vi "Initialize.vi"(5 "TCP Configuration":T1, 7 "Serial Port":refnum<visa-resource-name>="N/A", 8 "Error In":errorcluster, 10 "Interface":T2, 11 "Platform":T7) -> (0 "Error Out":errorcluster, 2 "Device Name":string, 3 "LINX Ref":T3)   [LabVIEW 2013, in "LVH-LINX.lvlib"]
doc: "Initialize a connection to a LINX device."
uses:
  <vilib>/LabVIEW Hacker/LINX/LVH-LINX.lvlib
  <vilib>/LabVIEW Hacker/LINX/Private/Type Defs/User Platform.ctl
  <vilib>/LabVIEW Hacker/LINX/Private/Type Defs/LINX Ref.ctl
  <vilib>/LabVIEW Hacker/LINX/Private/Type Defs/Platform.ctl
  <vilib>/LabVIEW Hacker/LINX/Private/Type Defs/Interface.ctl
  <vilib>/LabVIEW Hacker/LINX/Private/Device/Type Defs/LINX Device Config.ctl
  <vilib>/LabVIEW Hacker/LINX/Private/Device/Type Defs/TCP Config.ctl
  <vilib>/LabVIEW Hacker/LINX/Private/Type Defs/Device Family.ctl
  <vilib>/LabVIEW Hacker/LINX/Private/Type Defs/Channel FGV States.ctl
  <vilib>/LabVIEW Hacker/LINX/Private/Device/Device.lvlib
  <vilib>/LabVIEW Hacker/LINX/Private/Type Defs/Devices - NI.ctl
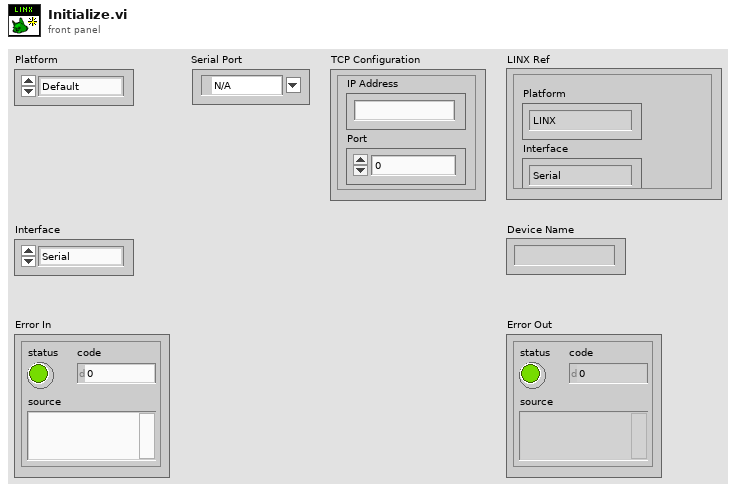
[diagram p1: front panel]
types:
  T1 = typedef "LVH-LINX.lvlib/Device.lvlib/TCP Config.ctl" = cluster{"IP Address":string, "Port":u16}
  T2 = typedef "LVH-LINX.lvlib/Interface.ctl" = enum16{"Serial", "TCP"}
  T3 = typedef "LVH-LINX.lvlib/LINX Ref.ctl" = cluster{"Platform":T4, "Interface":T2, "LINX Device Config":T5}
  T4 = typedef "LVH-LINX.lvlib/Platform.ctl" = enum16{"LINX", "myRIO"}
  T5 = typedef "LVH-LINX.lvlib/Device.lvlib/LINX Device Config.ctl" = cluster{"Interface":T2, "COM Port":refnum<visa-resource-name>, "TCP Configuration":T1, "Device Family":T6, "Device ID":u8, "Device Name":string, "TCP Ref":refnum<k5>}
  T6 = typedef "LVH-LINX.lvlib/Device Family.ctl" = enum8{"National Instruments", "Digilent", "Arduino"}
  T7 = typedef "LVH-LINX.lvlib/User Platform.ctl" = enum16{"Default", "LINX", "myRIO"}
  T8 = typedef "LVH-LINX.lvlib/Devices - NI.ctl" = enum16{"myRIO-1900", "myRIO-1950"}
  T9 = typedef "LVH-LINX.lvlib/Channel FGV States.ctl" = enum16{"Initialize", "Get", "Set"}
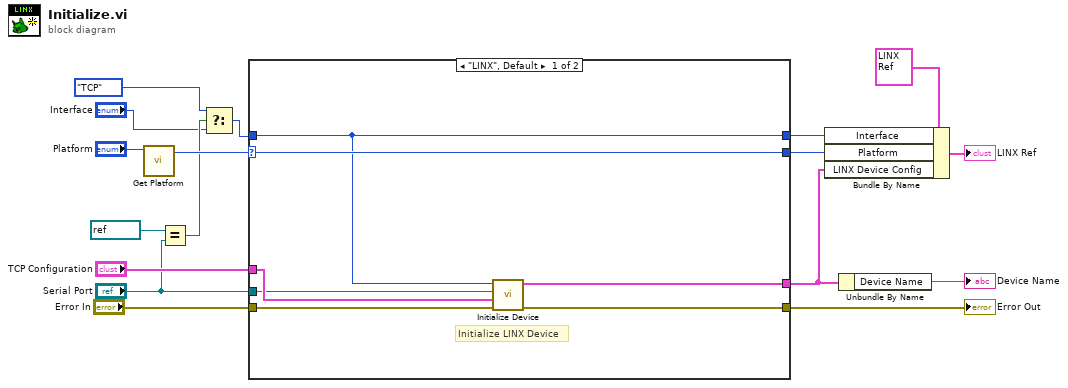
[diagram p0: block diagram]
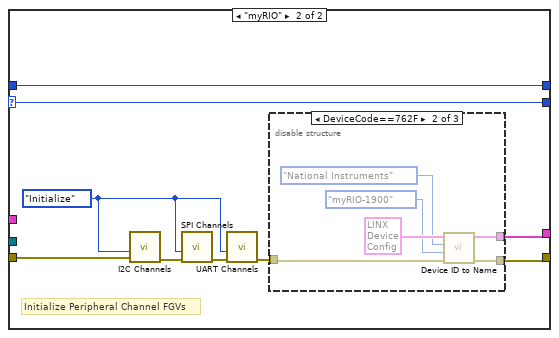
[diagram p2: hidden frame]
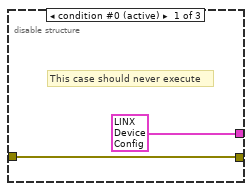
[diagram p3: hidden frame]
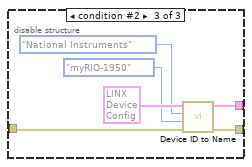
[diagram p4: hidden frame]
diagram:
  n1 = call <vilib>:"Get Platform.vi"("Platform"="Platform") -> ("Platform"=w15:T4)  [unwired: 10 in]
  n2 = Equal?(x=refnum<visa-resource-name> "N/A", y="Serial Port") -> (x = y?=w4:bool)
  n3 = Select(t=Interface."TCP" ("f"), s=w4, f="Interface") -> (s? t:f=w3:T2)
  n4 = case shown="\"LINX\", Default" w15 {
    selector: w15 -> [w24 w33]
    tunnel: [w21 w30] -> w8
    tunnel: [w22 w29] -> w13
    tunnel: "Error In" -> [w23 w31]
    tunnel: [w24 w33] -> w10
    tunnel: "Serial Port" -> [w19 _]
    tunnel: w3 -> [w18 w32]
    tunnel: "TCP Configuration" -> [w20 _]
    tunnel: [w18 w32] -> w9
    frame "LINX", Default {
      # "Initialize LINX Device"
      n5 = call <vilib>:"Initialize Device.vi"("Error In"=w23, "TCP Configuration"=w20, "COM Port"=w19, "Interface"=w18) -> ("Error Out"=w22:errorcluster, "LINX Device Config"=w21:T5)  [unwired: 5 in, 1 out]
    }
    frame "myRIO" {
      w25 = Channel_FGV_States."Initialize" ("Channel State")
      # "Initialize Peripheral Channel FGVs"
      n6 = call <vilib>:"I2C Channels.vi"("Error In"=w31, "Channel State"=w25) -> ("Error Out"=w28:errorcluster)  [unwired: 8 in, 1 out]
      n7 = call <vilib>:"SPI Channels.vi"("Error In"=w28, "Channel State"=w25) -> ("Error Out"=w27:errorcluster)  [unwired: 8 in, 1 out]
      n8 = call <vilib>:"UART Channels.vi"("Error In"=w27, "Channel State"=w25) -> ("Error Out"=w26:errorcluster)  [unwired: 8 in, 1 out]
      n9 = disable-structure shown="DeviceCode==762F" {
        disable-tunnel: w26 -> [w35 w41 w47]
        disable-tunnel: [T5 {"Interface"=enum."Serial", "COM Port"="", "TCP Configuration"={"IP Address"="", "Port"=0}, "Device Family"=enum."National Instruments", "Device ID"=0, "Device Name"="", "TCP Ref"=refnum} ("LINX Device Config") w38 w44] -> w30
        disable-tunnel: [w35 w37 w43] -> w29
        frame condition #0 (active) {
          # "This case should never execute"
        }
        frame condition #1 {
          n10 = call <vilib>:"Device ID to Name.vi"("Error In"=w41, "Device ID"=Devices_-_NI."myRIO-1900" ("NI Device"), "Device Family"=Device_Family."National Instruments", "LINX Device Config"=T5 {"Interface"=enum."Serial", "COM Port"="", "TCP Configuration"={"IP Address"="", "Port"=0}, "Device Family"=enum."National Instruments", "Device ID"=0, "Device Name"="", "TCP Ref"=refnum}) -> ("Error Out"=w37:errorcluster, "LINX Device Config"=w38:T5)  [unwired: 5 in, 1 out]
        }
        frame condition #2 {
          n11 = call <vilib>:"Device ID to Name.vi"("Error In"=w47, "Device ID"=Devices_-_NI."myRIO-1950" ("NI Device"), "Device Family"=Device_Family."National Instruments", "LINX Device Config"=T5 {"Interface"=enum."Serial", "COM Port"="", "TCP Configuration"={"IP Address"="", "Port"=0}, "Device Family"=enum."National Instruments", "Device ID"=0, "Device Name"="", "TCP Ref"=refnum}) -> ("Error Out"=w43:errorcluster, "LINX Device Config"=w44:T5)  [unwired: 5 in, 1 out]
        }
      }
    }
  }
  "Error Out" <- w13
  n12 = Bundle By Name(cluster=T3 {"Platform"=enum."LINX", "Interface"=enum."Serial", "LINX Device Config"={"Interface"=enum."Serial", "COM Port"="", "TCP Configuration"={"IP Address"="", "Port"=0}, "Device Family"=enum."National Instruments", "Device ID"=0, "Device Name"="", "TCP Ref"=refnum}} ("LINX Resource"), "Interface"=w9, "Platform"=w10, "LINX Device Config"=w8) -> (→"LINX Ref":T3)
  n13 = Unbundle By Name(w8) -> ("Device Name"=→"Device Name":string)
